vi "DIO (B).vi"(8 "error in (no error)":errorcluster, 10 "Write":u8, 11 "DIO":refnum<k24>) -> (0 "error out":errorcluster, 3 "Read":u8)   [LabVIEW 2011]
doc: "Control the digital input/output port with binary constant values(basic version)."
uses:
  C:/Program Files/Metrohm Autolab/Autolab SDK 1.10/EcoChemie.Autolab.Sdk.dll
  EcoChemie.Autolab.Sdk.dll
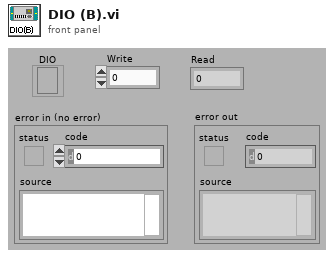
[diagram p1: front panel]
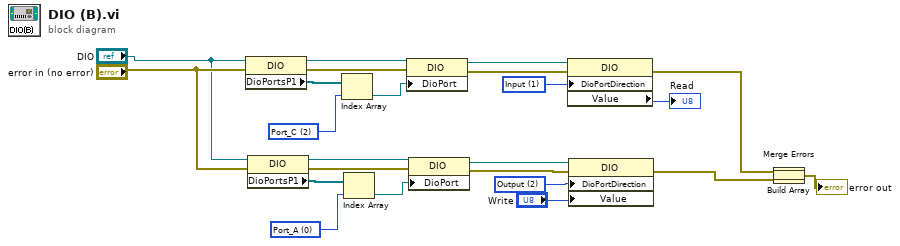
[diagram p0: block diagram]
diagram:
  w9 = 0 items=["Port_A", "Port_B", "Port_C"] ("Port P1 2")
  w20 = 2 items=["Port_A", "Port_B", "Port_C"] ("Port P1")
  w16 = u8 2 items=["Input"=1, "Output"=2] ("DioPortDirection")
  w17 = u8 1 items=["Input"=1, "Output"=2] ("DioPortDirection")
  n1 = property class="DIO"(reference="DIO", error in="error in (no error)") -> (reference out=w24:refnum<k24>, error out=w23:errorcluster, "DioPortsP1"=w21:refnum<k24>[])
  n2 = property class="DIO"(reference="DIO", error in="error in (no error)") -> (reference out=w13:refnum<k24>, error out=w12:errorcluster, "DioPortsP1"=w10:refnum<k24>[])
  n3 = Index Array(array=w21, index=w20) -> (element=w22:refnum<k24>)
  n4 = Index Array(array=w10, index=w9) -> (element=w11:refnum<k24>)
  n5 = property class="DIO"(reference=w24, error in=w23, "DioPort"=w22) -> (reference out=w15:refnum<k24>, error out=w14:errorcluster)
  n6 = property class="DIO"(reference=w13, error in=w12, "DioPort"=w11) -> (reference out=w8:refnum<k24>, error out=w7:errorcluster)
  n7 = property class="DIO"(reference=w15, error in=w14, "DioPortDirection"=w17) -> (error out=w19:errorcluster, "Value"=→"Read":u8)  [unwired: 1 out]
  n8 = property class="DIO"(reference=w8, error in=w7, "DioPortDirection"=w16, "Value"="Write") -> (error out=w5:errorcluster)  [unwired: 1 out]
  n9 = Build Array(w19, w5) -> (w1:errorcluster[])
  n10 = Merge Errors(w1) -> (→"error out":errorcluster)
